vi "Prepare New Cycle.vi"(8 "error in (no error)":errorcluster, 11 "Response Synchronizer in":refnum<class "Response Synchronizer.lvclass">) -> (0 "error out":errorcluster, 3 "Response Synchronizer out":refnum<class "Response Synchronizer.lvclass">)   [LabVIEW 2021, in "Response Synchronizer.lvclass"]
uses:
  Response Synchronizer.lvclass
  NHMFL_Core/Libraries/Instruments/Results/Acquired Result/Acquired Result.lvclass
  Response Synchronizer.lvclass/Response Synchronizer.ctl
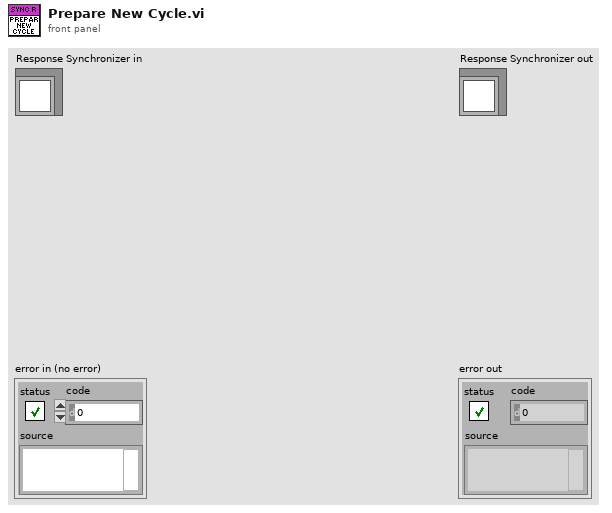
[diagram p1: front panel]
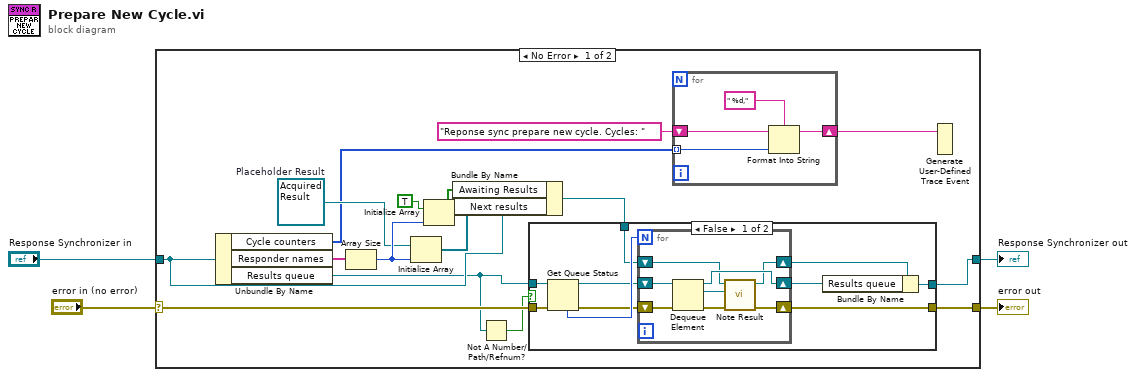
[diagram p0: block diagram]
diagram:
  n1 = case shown="No Error" "error in (no error)" {
    selector: "error in (no error)" -> [w11 w46]
    tunnel: [w10 w46] -> w3
    tunnel: [w12 w45] -> w1
    tunnel: "Response Synchronizer in" -> [w14 w45]
    frame No Error {
      w17 = refnum<class "Acquired Result.lvclass"> refnum  # Placeholder Result
      n2 = Unbundle By Name(w14) -> ("Cycle counters"=w7:i32[], "Responder names"=w15:string[], "Results queue"=w6:refnum<queue>)
      n3 = Array Size(array=w15) -> (size(s)=w20:i32)
      n4 = Initialize Array(w17, w20) -> (w19:refnum<class "Acquired Result.lvclass">[])
      n5 = Initialize Array(TRUE, w20) -> (w18:bool[])
      n6 = Bundle By Name(cluster=w14, "Awaiting Results"=w18, "Next results"=w19) -> (w13:refnum<class "Response Synchronizer.lvclass">)
      n7 = Not A Number/Path/Refnum?(number/path/refnum=w6) -> (NaN/Path/Refnum?=w5:bool)
      n8 = case shown="False" w5 {
        tunnel: w6 -> [w30 _]
        tunnel: w13 -> [w27 w39]
        tunnel: [w25 w39] -> w12
        tunnel: w11 -> [w22 w40]
        tunnel: [w21 w40] -> w10
        frame False {
          n9 = Get Queue Status(queue=w30, error in (no error)=w22) -> (queue out=w28:refnum<queue>, error out=w23:errorcluster, # elements in queue=w29:i32)  [unwired: 1 in, 5 out]
          n10 = for {
            N: w29 -> [_]
            shift-right: [w37] -> w24
            shift-left: w28 -> [w38]
            shift-right: [w35] -> w26
            shift-left: w27 -> [w36]
            shift-right: [w33] -> w21
            shift-left: w23 -> [w32]
            n11 = Dequeue Element(queue=w38, error in (no error)=w32) -> (queue out=w37:refnum<queue>, element=w31:refnum<class "Acquired Result.lvclass">, error out=w34:errorcluster)  [unwired: 1 in, 1 out]
            n12 = call-dynamic "Note Result.vi"("error in (no error)"=w34, "Acquired Result.lvclass"=w31, "Response Synchronizer in"=w36) -> ("error out"=w33:errorcluster, "Response Synchronizer out"=w35:refnum<class "Response Synchronizer.lvclass">)  [unwired: 7 in]
          }
          n13 = Bundle By Name(cluster=w26, "Results queue"=w24) -> (w25:refnum<class "Response Synchronizer.lvclass">)
        }
        frame True {
        }
      }
      n14 = for {
        tunnel: w7 -> [w44] mode=indexing
        shift-right: [w41] -> w8
        shift-left: "Reponse sync prepare new cycle. Cycles: " ("format string") -> [w43]
        n15 = Format Into String(format string=" %d,", initial string=w43, w44) -> (resulting string=w41:string)  [unwired: 1 in, 1 out]
      }
      n16 = Generate User-Defined Trace Event(2:w8) -> ()  [unwired: 1 in]
    }
    frame Error {
    }
  }
  "error out" <- w3
  "Response Synchronizer out" <- w1
